vi "write TBM configuration.vi"(8 "error in":errorcluster, 10 "configuration":refnum<class "TBM configuration.lvclass">, 11 "tag bus processing plugin editor node in":refnum<class "tag bus processing plugin editor node.lvclass">) -> (0 "error out":errorcluster, 3 "tag bus processing plugin editor node out":refnum<class "tag bus processing plugin editor node.lvclass">)   [LabVIEW 2013, in "tag bus processing plugin editor node.lvclass"]
uses:
  tag bus processing plugin editor node.lvclass
  <vilib>/NI/Tag Bus Module Framework/root configuration/TBM configuration.lvclass
  module/configuration/tag bus processing plugin module configuration.lvclass
  tag bus processing plugin editor node.lvclass/tag bus processing plugin editor node.ctl
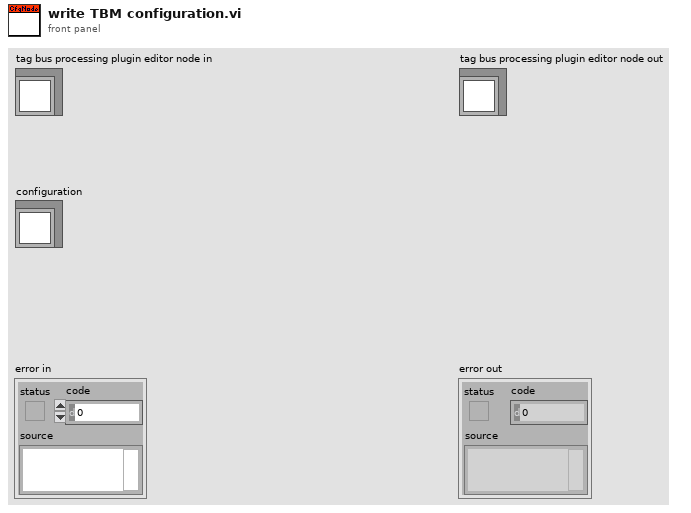
[diagram p1: front panel]
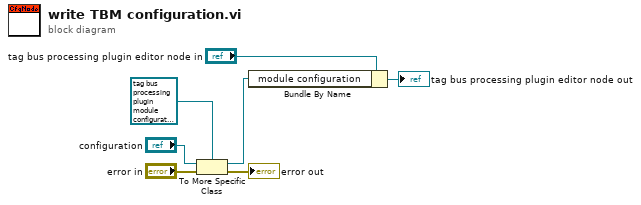
[diagram p0: block diagram]
diagram:
  n1 = To More Specific Class(target class=refnum<class "tag bus processing plugin module configuration.lvclass"> refnum ("module configuration"), reference="configuration", error in="error in") -> (specific class reference=w3:refnum<class "tag bus processing plugin module configuration.lvclass">, error out=→"error out":errorcluster)
  n2 = Bundle By Name(cluster="tag bus processing plugin editor node in", "module configuration"=w3) -> (→"tag bus processing plugin editor node out":refnum<class "tag bus processing plugin editor node.lvclass">)
